vi "Find Average Center Setup.vi"(4 "Sensor Thickness":dbl, 6 "Assembly Type":string, 8 "Position":i32, 9 "Tray Number":i32, 10 "XYZTheta":dbl[](array[numeric]), 11 "Component":T1) -> (3 "output cluster":T1)   [LabVIEW 2021, in "Component Tray.lvclass"]
uses:
  Component Tray.lvclass
  Find Component.ctl
  Controller/Camera/Machine Vision.ctl
  Controller/Camera/Camera.lvclass
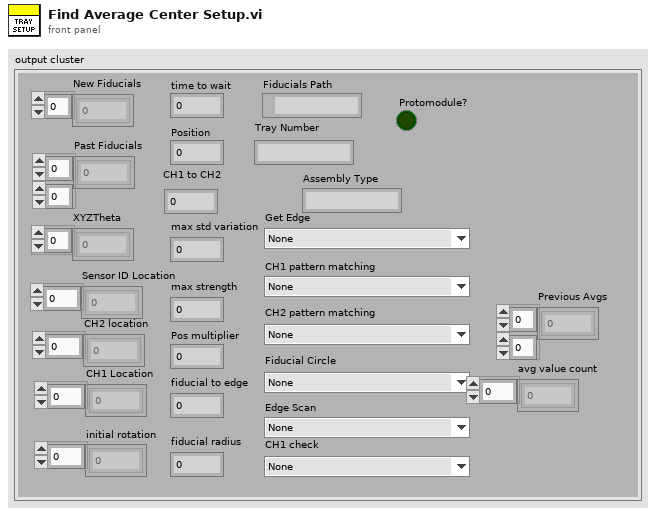
[diagram p1: front panel]
types:
  T1 = typedef "Component Tray.lvclass/Find Component.ctl" = cluster{"New Fiducials":dbl[], "Past Fiducials":dbl[][], "XYZTheta":dbl[], "Fiducials Path":path, "Position":i32, "CH1 Location":dbl[], "Sensor ID Location":dbl[], "initial rotation":dbl[], "CH2 location":dbl[], "max std variation":dbl, "max strength":dbl, "CH2 pattern matching":T2, "Fiducial Circle":T2, "Get Edge":T2, "Pos multiplier":dbl, "time to wait":u32, "fiducial to edge":dbl, "Protomodule?":bool, "Assembly Type":string, "CH1 to CH2":dbl, "Tray Number":string, "fiducial radius":dbl, "4 fiducials?":bool, "CH1 check":T2, "Edge Scan":T2, "CH1 pattern matching":T2, "Sensor Thickness":dbl, "Previous Avgs":dbl[][], "avg value count":dbl[]}
  T2 = typedef "Camera.lvclass/Machine Vision.ctl" = enum16{"None", "Assembly Tray Circle", "Assembly Tray Fiducial", "Partial Hexaboard", "sensor edge init", "HB edge init", "sensor edge pos1", "sensor edge pos2", "HB edge pos1", "HB edge pos2", "Sensor CH1-2", "HB CH1", "HB CH2", "V3 Sensor Circle", "Hexaboard Circle", "sensor CH1 check", "HB CH1 check ", "sensor ID"}
  T3 = typedef "File Paths.ctl" = cluster{"Glue Pattern Folder":path, "Carrier Tray Folder":path, "Pick Up Tool Fixture Folder":path, "Components Folder":path, "Bellows Tool Offset.txt":path, "Pick Up Tool Offset.txt":path, "Dispense Tip Offset.txt":path, "Log Files":path, "Gantry Assembly Map.txt":path, "Syringe and offset map.txt":path, "Controllers Folder":path, "Local dbase config":path}
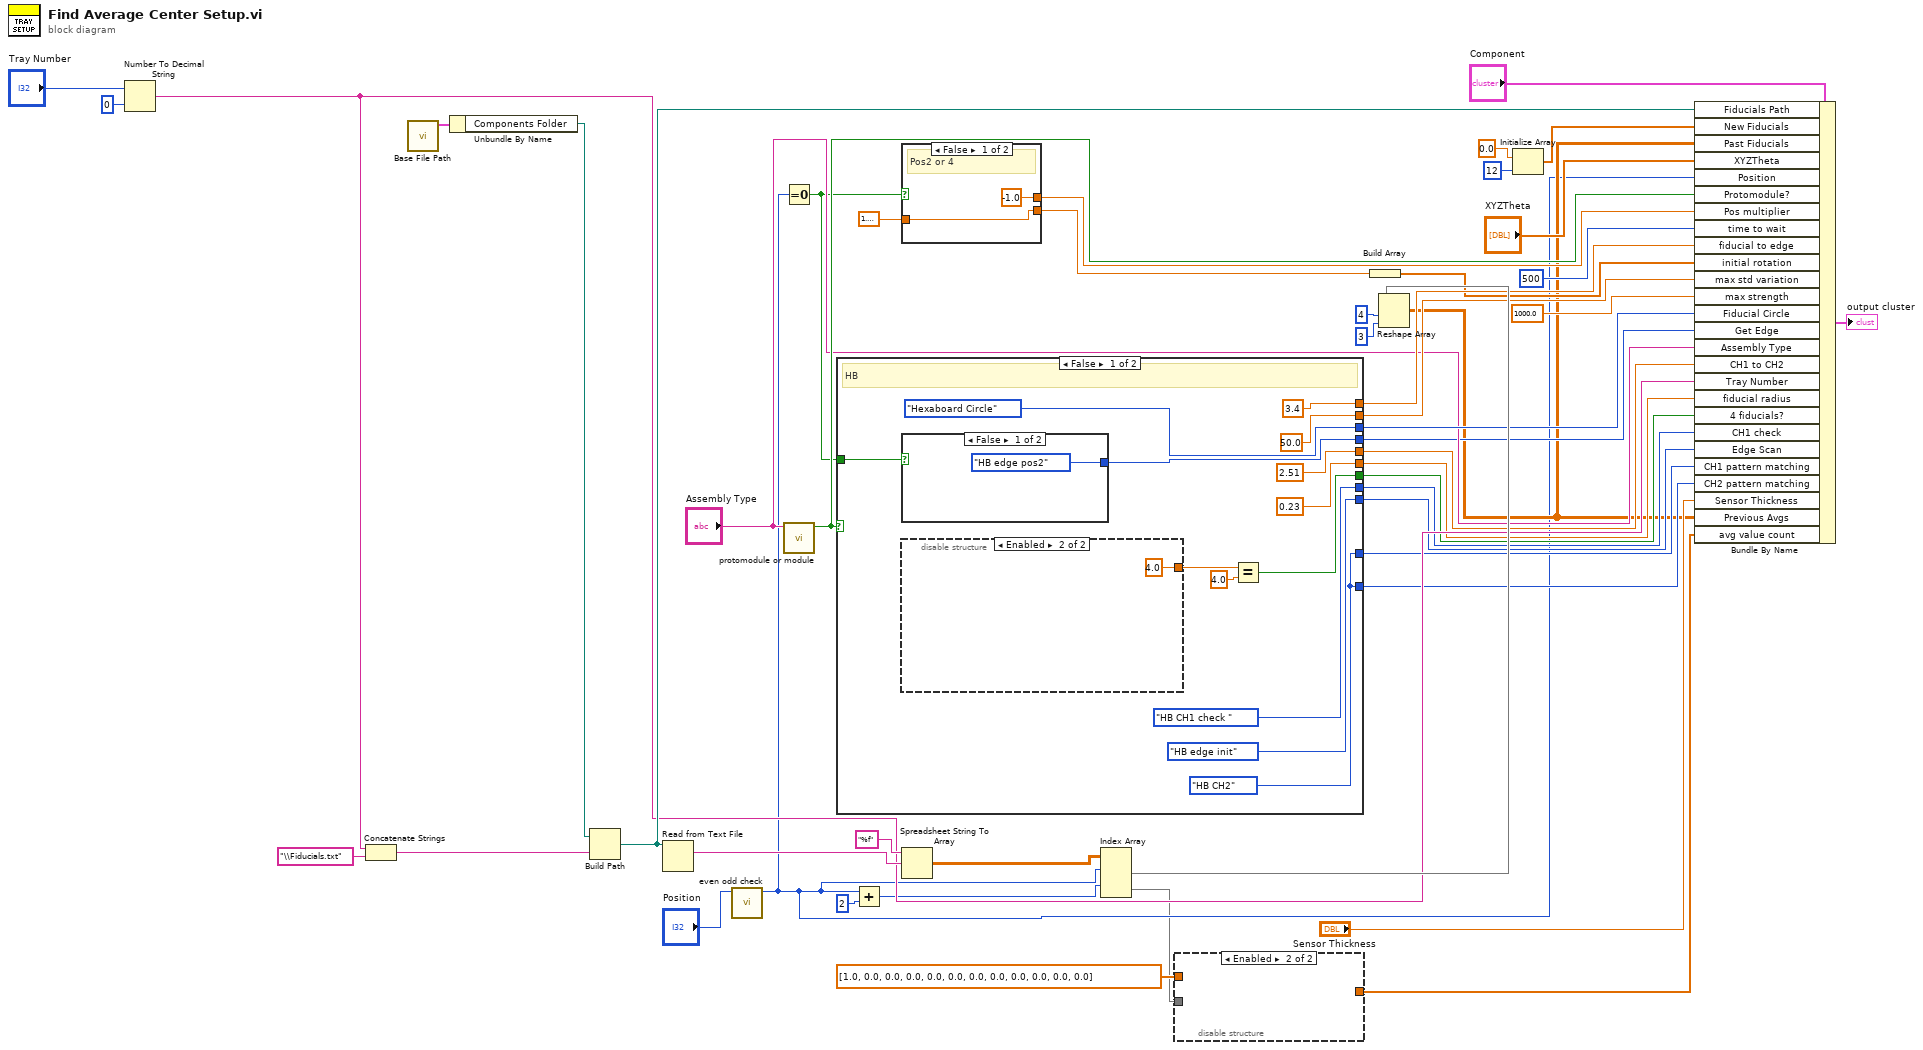
[diagram p0: block diagram]
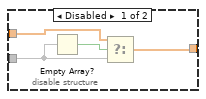
[diagram p2: hidden frame]
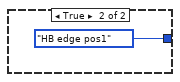
[diagram p3: hidden frame]
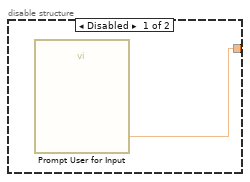
[diagram p4: hidden frame]
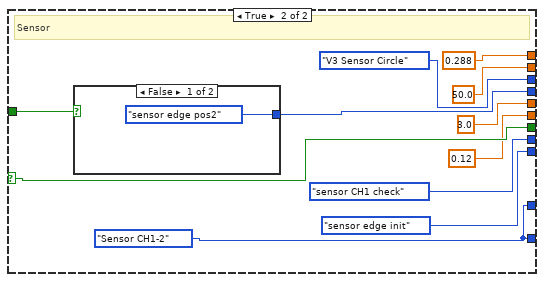
[diagram p5: hidden frame]
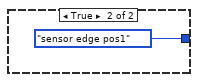
[diagram p6: hidden frame]
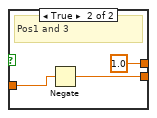
[diagram p7: hidden frame]
diagram:
  n1 = Number To Decimal String(number="Tray Number", width (-)=i16 0) -> (decimal integer string=w18:string)
  n2 = Concatenate Strings "Concatenate Strings"(w18, "\\Fiducials.txt" ("string")) -> (w47:string)
  n3 = call "Base File Path.vi"() -> ("Paths Out"=w43:T3)  [unwired: 11 in]
  n4 = Unbundle By Name(w43) -> ("Components Folder"=w48:path)
  n5 = Build Path(base path=w48, name or relative path=w47) -> (appended path=w44:path)
  n6 = Read from Text File(file (use dialog)=w44) -> (text=w42:string)  [unwired: 3 in, 3 out]
  n7 = call "even odd check.vi"("position"="Position") -> ("index"=w6:i32)  [unwired: 10 in]
  n8 = Equal To 0?(x=w6) -> (x = 0?=w14:bool)
  n9 = call "protomodule or module.vi"("assembly type"="Assembly Type") -> ("protomodule? (T)"=w27:bool)  [unwired: 10 in]
  n10 = case shown="False" w27 {
    selector: w27 -> [_ w73]
    tunnel: [3.4 ("fiducial to edge") 0.288 ("fiducial to edge")] -> w26
    tunnel: [w50 w68] -> w11
    tunnel: [Machine_Vision."Hexaboard Circle" ("Fiducial Circle") Machine_Vision."V3 Sensor Circle" ("Fiducial Circle")] -> w22
    tunnel: [50.0 ("max std variation") 50.0 ("max std variation")] -> w21
    tunnel: [2.51 ("CH1 to CH2") 3.0 ("CH1 to CH2")] -> w19
    tunnel: [w57 w73] -> w17
    tunnel: [Machine_Vision."HB CH1 check " ("CH1 check") Machine_Vision."sensor CH1 check" ("CH1 check")] -> w16
    tunnel: [0.23 ("fiducial radius") 0.12 ("fiducial radius")] -> w15
    tunnel: w14 -> [w54 w70]
    tunnel: [w53 w69] -> w13
    tunnel: [w50 w68] -> w12
    tunnel: [Machine_Vision."HB edge init" ("Edge Scan") Machine_Vision."sensor edge init" ("Edge Scan")] -> w10
    frame False {
      w50 = Machine_Vision."HB CH2" ("Pattern Matching")
      # "HB"
      n11 = case shown="False" w54 {
        tunnel: [Machine_Vision."HB edge pos2" ("Initial Edge") Machine_Vision."HB edge pos1" ("Initial Edge")] -> w53
        frame False {
        }
        frame True {
        }
      }
      n12 = disable-structure shown="Enabled" {
        disable-tunnel: [w65 4.0 ("NumFD")] -> w59
        frame Disabled {
          n13 = call "Prompt User for Input"() -> ("NumFD"=w65:dbl)  [unwired: 17 in, 2 out]
        }
        frame Enabled {
        }
      }
      n14 = Equal?(x=w59, y=4.0) -> (x = y?=w57:bool)
    }
    frame True {
      w68 = Machine_Vision."Sensor CH1-2" ("Pattern Matching")
      # "Sensor"
      n15 = case shown="False" w70 {
        tunnel: [Machine_Vision."sensor edge pos2" ("Initial Edge") Machine_Vision."sensor edge pos1" ("Initial Edge")] -> w69
        frame False {
        }
        frame True {
        }
      }
    }
  }
  n16 = Add(x=w6, y=2) -> (x+y=w4:i32)
  n17 = case shown="False" w14 {
    tunnel: [-1.0 ("Pos multiplier") 1.0 ("Pos multiplier")] -> w29
    tunnel: 1.5707963267948966 -> [w80 w83]
    tunnel: [w80 w82] -> w23
    frame False {
      # "Pos2 or 4"
    }
    frame True {
      # "Pos1 and 3"
      n18 = Negate(x=w83) -> (-x=w82:dbl)
    }
  }
  n19 = Spreadsheet String To Array(format string="%f", spreadsheet string=w42) -> (array=w40:dbl[][])  [unwired: 2 in]
  n20 = Index Array "Index Array"(array=w40, index (row) #1=w6, index (row) #2=w4) -> (element #1=w39:dbl[], element #2=w2:dbl[])  [unwired: 2 in]
  n21 = disable-structure shown="Enabled" {
    disable-tunnel: dbl[] [1.0, 0.0, 0.0, 0.0, 0.0, 0.0, 0.0, 0.0, 0.0, 0.0, 0.0, 0.0] ("t") -> [w87 _]
    disable-tunnel: w2 -> [w86 _]
    disable-tunnel: [w85 _] -> w1
    frame Disabled {
      n22 = Empty Array?(array=w86) -> (empty?=w88:bool)
      n23 = Select(t=w87, s=w88, f=w86) -> (s? t:f=w85:dbl[])
    }
    frame Enabled {
    }
  }
  n24 = Build Array(w23) -> (w25:dbl[])
  n25 = Reshape Array(w39, 4 ("dimension size"), 3 ("dimension size")) -> (w7:dbl[][])
  n26 = Initialize Array(0.0 ("element"), 12 ("dimension size")) -> (w33:dbl[])
  n27 = Bundle By Name "Bundle By Name"(cluster="Component", "Fiducials Path"=w44, "New Fiducials"=w33, "Past Fiducials"=w7, "XYZTheta"="XYZTheta", "Position"=w6, "Protomodule?"=w27, "Pos multiplier"=w29, "time to wait"=u32 500, "fiducial to edge"=w26, "initial rotation"=w25, "max std variation"=w21, "max strength"=1000.0, "Fiducial Circle"=w22, "Get Edge"=w13, "Assembly Type"="Assembly Type", "CH1 to CH2"=w19, "Tray Number"=w18, "fiducial radius"=w15, "4 fiducials?"=w17, "CH1 check"=w16, "Edge Scan"=w10, "CH1 pattern matching"=w12, "CH2 pattern matching"=w11, "Sensor Thickness"="Sensor Thickness", "Previous Avgs"=w7, "avg value count"=w1) -> (→"output cluster":T1)
